vi "main.vi"() -> ()   [LabVIEW 2024]
uses:
  Message_t.ctl
  <vilib>/addons/_JKI.lib/REST Client/classes/REST Client/REST Client.lvclass
  MeasurementJson_t.ctl
  HealthJson_t.ctl
panel:
  out "Status":bool
  out "Response":string
  out "Response":string
  in  "Base URL":string(combo)
  in  "PredefinedURL":bool
  in  "auto read":bool
  out "Waveform Graph 2":dbl[](graph)
  in  "Custom URL":string
  in  "connect":bool
  in  "measure":bool
  in  "exit":bool
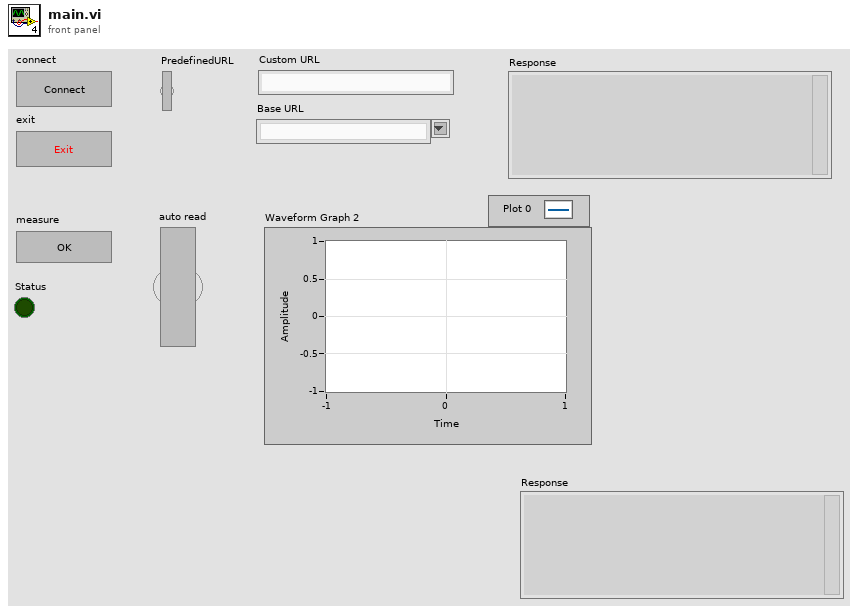
[diagram p1: front panel]
types:
  T1 = cluster{"polaczenie":refnum<class "REST Client.lvclass">, "dane":dbl[], "healthy":bool, "text":string}
  T2 = typedef "Message_t.ctl" = cluster{"action":enum16{"CheckHealth", "GetMeasurement", "ExitProgram", "OpenSession", "CloseSession", "SetFlag"}, "parameters":variant}
  T3 = typedef "MeasurementJson_t.ctl" = cluster{"id":i64, "sensor_id":string, "value":dbl, "unit":string}
  T4 = typedef "HealthJson_t.ctl" = cluster{"status":string}
  T5 = enum16{"CheckHealth", "GetMeasurement", "ExitProgram", "OpenSession", "CloseSession", "SetFlag"}
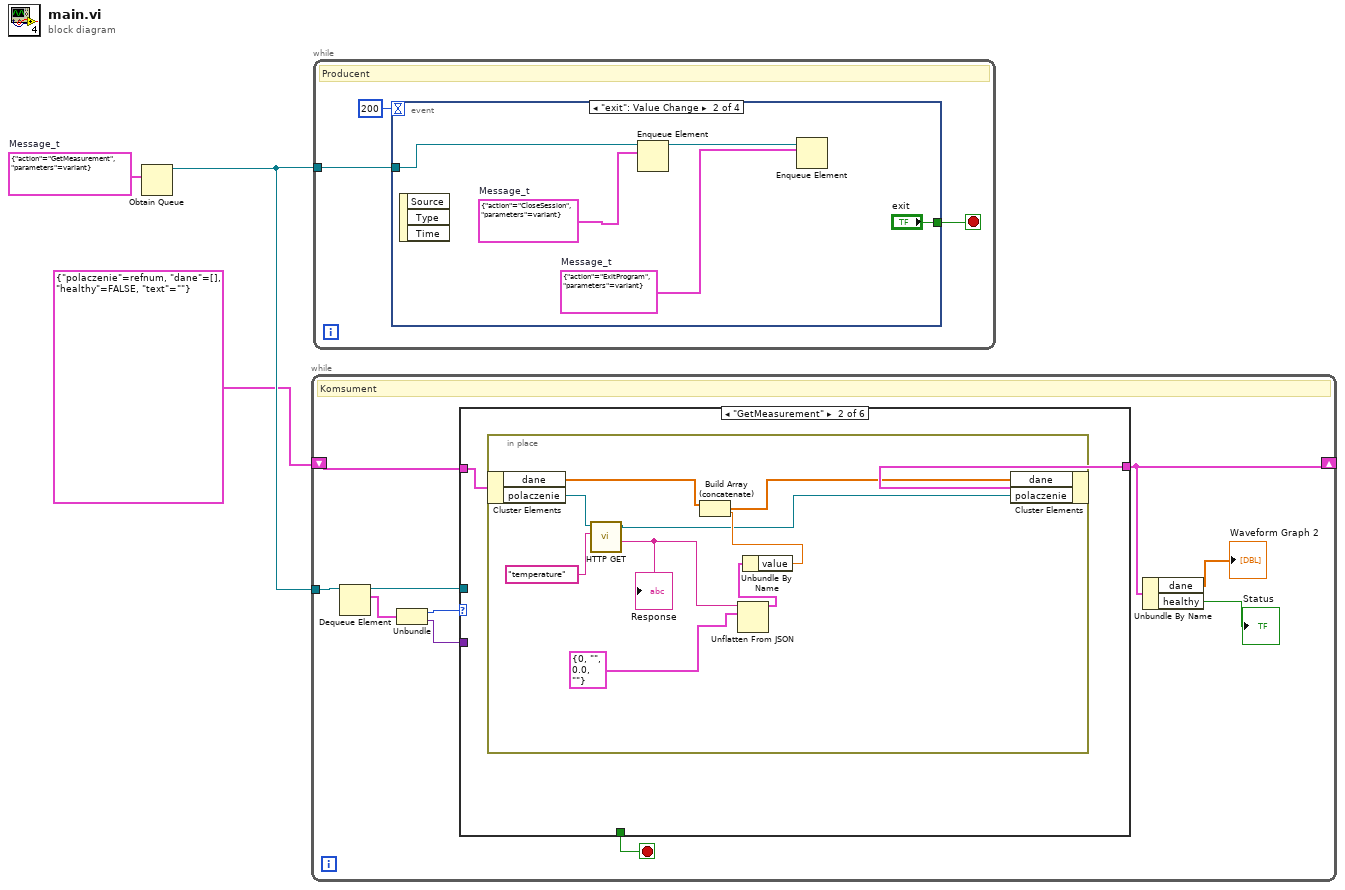
[diagram p0: block diagram]
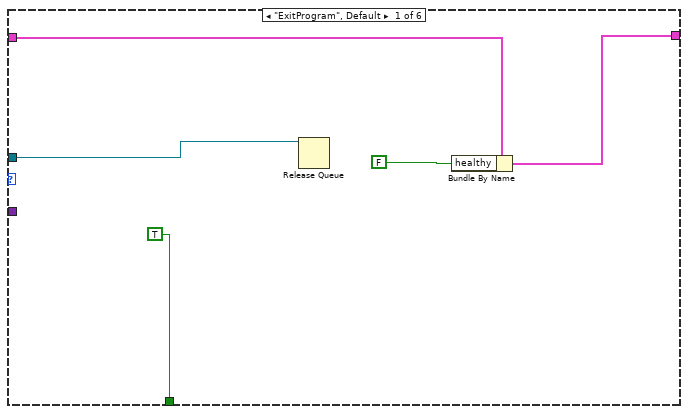
[diagram p2: hidden frame]
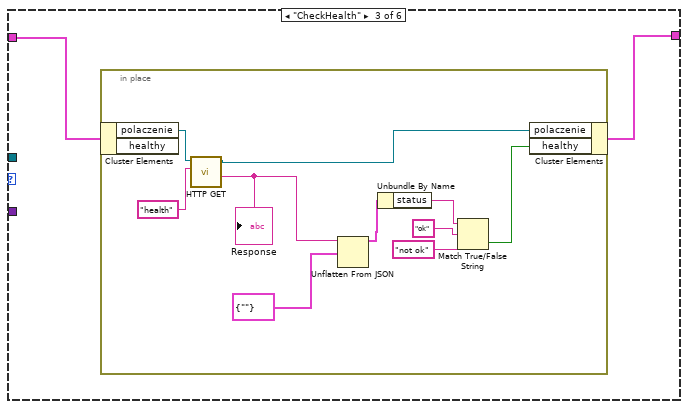
[diagram p3: hidden frame]
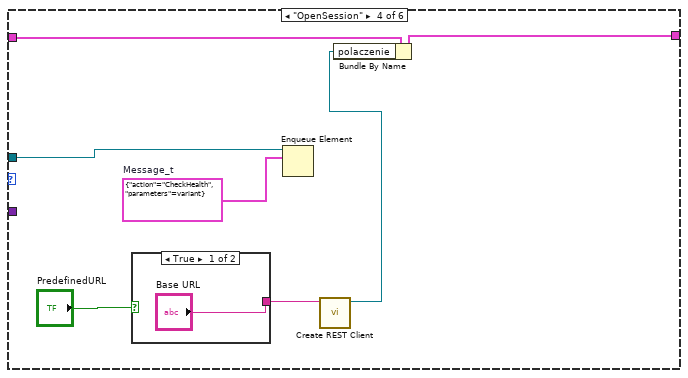
[diagram p4: hidden frame]
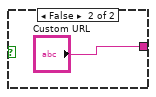
[diagram p5: hidden frame]
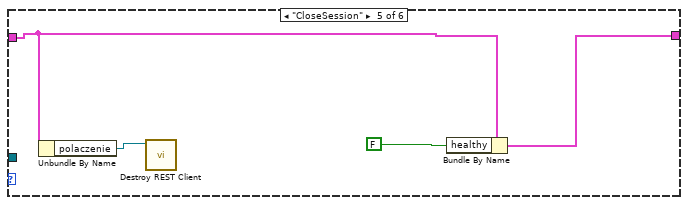
[diagram p6: hidden frame]
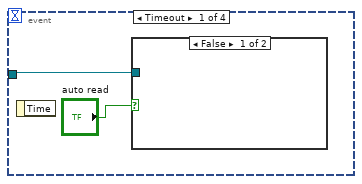
[diagram p8: hidden frame]
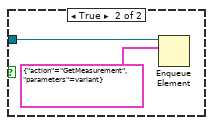
[diagram p9: hidden frame]
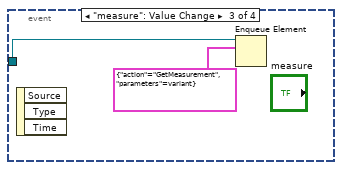
[diagram p10: hidden frame]
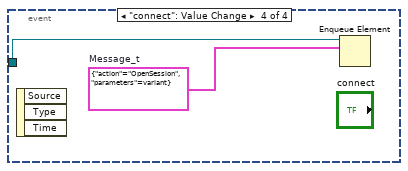
[diagram p11: hidden frame]
diagram:
  w2 = T2 {"action"=enum."GetMeasurement", "parameters"=variant}  # Message_t
  n1 = Obtain Queue(element data type=w2) -> (queue out=w3:refnum<queue>)  [unwired: 4 in, 2 out]
  n2 = while {
    tunnel: w3 -> [w13]
    shift-right: [w6] -> _
    shift-left: T1 {"polaczenie"=refnum, "dane"=[], "healthy"=FALSE, "text"=""} -> [w7]
    stop <- w8 stop-if-true
    # "Komsument"
    n3 = Dequeue Element(queue=w13) -> (queue out=w9:refnum<queue>, element=w12:T2)  [unwired: 2 in, 2 out]
    n4 = Unbundle(w12) -> ("action"=w11:T5, "parameters"=w10:variant)
    n5 = case shown="\"GetMeasurement\"" w11 {
      tunnel: w10 -> [_ _ _ _ _ _]
      tunnel: w9 -> [w18 _ _ w42 _ _]
      tunnel: [TRUE _ _ _ _ _] -> w8
      tunnel: w7 -> [w15 w20 w31 w48 w53 w55]
      tunnel: [w14 w19 w30 w47 w51 w55] -> w6
      frame "ExitProgram", Default {
        n6 = Release Queue(queue=w18) -> ()  [unwired: 2 in, 3 out]
        n7 = Bundle By Name(cluster=w15, "healthy"=FALSE) -> (w14:T1)
      }
      frame "GetMeasurement" {
        n8 = in-place "In Place Element Structure" {
          n9 = in-place-cluster #1(w20) -> ("dane"=w25:dbl[], "polaczenie"=w23:refnum<class "REST Client.lvclass">)
          n10 = call-dynamic "HTTP GET.vi"("Path"="temperature", "REST Client in"=w23) -> ("Response body"=w29:string, "REST Client out"=w22:refnum<class "REST Client.lvclass">)  [unwired: 4 in, 4 out]
          "Response" <- w29
          n11 = Unflatten From JSON(JSON string=w29, type and defaults=T3 {"id"=0, "sensor_id"="", "value"=0.0, "unit"=""} ("Cluster")) -> (value=w28:T3)  [unwired: 5 in, 1 out]
          n12 = Unbundle By Name(w28) -> ("value"=w27:dbl)
          n13 = Build Array (concatenate)(w25, w27) -> (w24:dbl[])
          n14 = in-place-cluster #1("dane"=w24, "polaczenie"=w22) -> (w19:T1)
        }
      }
      frame "CheckHealth" {
        n15 = in-place "In Place Element Structure" {
          n16 = in-place-cluster #2(w31) -> ("polaczenie"=w38:refnum<class "REST Client.lvclass">)  [unwired: 1 out]
          n17 = call-dynamic "HTTP GET.vi"("Path"="health", "REST Client in"=w38) -> ("Response body"=w41:string, "REST Client out"=w37:refnum<class "REST Client.lvclass">)  [unwired: 4 in, 4 out]
          "Response" <- w41
          n18 = Unflatten From JSON(JSON string=w41, type and defaults=T4 {"status"=""} ("Cluster")) -> (value=w40:T4)  [unwired: 5 in, 1 out]
          n19 = Unbundle By Name(w40) -> ("status"=w35:string)
          n20 = Match True/False String(2:"not ok" ("false string"), 3:"ok" ("true string"), 4:w35) -> (0:w32:bool)  [unwired: 1 out]
          n21 = in-place-cluster #2("polaczenie"=w37, "healthy"=w32) -> (w30:T1)
        }
      }
      frame "OpenSession" {
        w43 = T2 {"action"=enum."CheckHealth", "parameters"=variant}  # Message_t
        n22 = case shown="True" "PredefinedURL" {
          tunnel: ["Base URL" "Custom URL"] -> w45
          frame True {
          }
          frame False {
          }
        }
        n23 = Enqueue Element(queue=w42, element=w43) -> ()  [unwired: 2 in, 3 out]
        n24 = call <vilib>:"Create REST Client.vi"("Base URL"=w45) -> ("REST Client out"=w44:refnum<class "REST Client.lvclass">)  [unwired: 9 in, 1 out]
        n25 = Bundle By Name(cluster=w48, "polaczenie"=w44) -> (w47:T1)
      }
      frame "CloseSession" {
        n26 = Unbundle By Name(w53) -> ("polaczenie"=w54:refnum<class "REST Client.lvclass">)
        n27 = call-dynamic "Destroy REST Client.vi"("REST Client in"=w54) -> ()  [unwired: 10 in, 1 out]
        n28 = Bundle By Name(cluster=w53, "healthy"=FALSE) -> (w51:T1)
      }
      frame "SetFlag" {
      }
    }
    n29 = Unbundle By Name(w6) -> ("dane"=→"Waveform Graph 2":dbl[], "healthy"=→"Status":bool)
  }
  n30 = while {
    tunnel: w3 -> [w58]
    stop <- w57 stop-if-true
    # "Producent"
    n31 = event shown="[1] \"exit\": Value Change" {
      selector: _ -> [_ _ _ _]
      dyn-events: _ -> [_ _ _ _]
      timeout: 200 -> [_ _ _ _]
      tunnel: w58 -> [w60 w67 w69 w71]
      tunnel: [_ "exit" _ _] -> w57
      event Timeout {
        n32 = event-data() -> ()  [unwired: 1 in, 1 out]
        n33 = case shown="False" "auto read" {
          tunnel: w60 -> [_ w62]
          frame False {
          }
          frame True {
            n34 = Enqueue Element(queue=w62, element=T2 {"action"=enum."GetMeasurement", "parameters"=variant}) -> ()  [unwired: 2 in, 3 out]
          }
        }
      }
      event "exit": Value Change {
        w63 = T2 {"action"=enum."CloseSession", "parameters"=variant}  # Message_t
        w64 = T2 {"action"=enum."ExitProgram", "parameters"=variant}  # Message_t
        n35 = event-data() -> ()  [unwired: 1 in, 3 out]
        n36 = Enqueue Element(queue=w67, element=w63) -> (queue out=w66:refnum<queue>)  [unwired: 2 in, 2 out]
        n37 = Enqueue Element(queue=w66, element=w64) -> ()  [unwired: 2 in, 3 out]
      }
      event "measure": Value Change {
        n38 = event-data() -> ()  [unwired: 1 in, 3 out]
        n39 = Enqueue Element(queue=w69, element=T2 {"action"=enum."GetMeasurement", "parameters"=variant}) -> ()  [unwired: 2 in, 3 out]
      }
      event "connect": Value Change {
        w70 = T2 {"action"=enum."OpenSession", "parameters"=variant}  # Message_t
        n40 = event-data() -> ()  [unwired: 1 in, 3 out]
        n41 = Enqueue Element(queue=w71, element=w70) -> ()  [unwired: 2 in, 3 out]
      }
    }
  }
